vi "List Info by Socket.vi"(7 "Socket":u32, 11 "LookupTable":refnum<data-value>) -> (3 "Pin Info":T1[](array[typedef]))   [LabVIEW 2024, in "Shared Steps.lvlib"]
doc: "Helper Routine: List all pins for a given socket."
uses:
  Shared Steps.lvlib
  Types/Pin Mapping.ctl
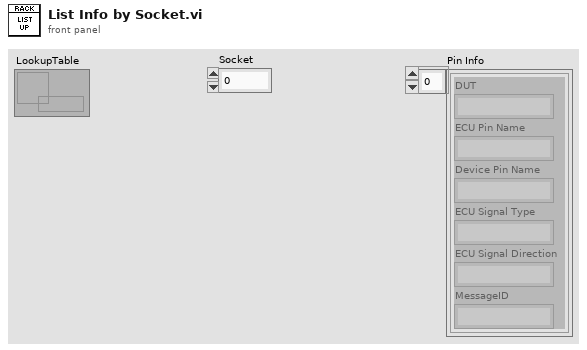
[diagram p1: front panel]
types:
  T1 = typedef "Shared Steps.lvlib/Pin Mapping.ctl" = cluster{"DUT":string, "ECU Pin Name":string, "Device Pin Name":string, "ECU Signal Type":string, "ECU Signal Direction":string, "MessageID":string}
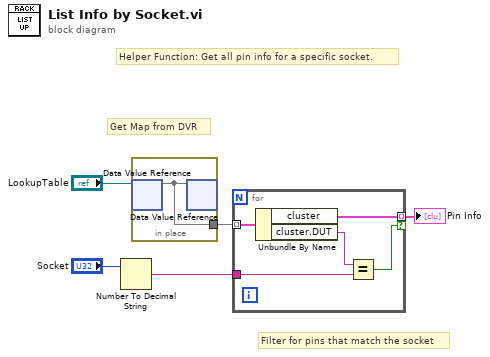
[diagram p0: block diagram]
diagram:
  # "Filter for pins that match the socket"
  # "Get Map from DVR"
  # "Helper Function: Get all pin info for a specific socket."
  n1 = Number To Decimal String(number="Socket") -> (decimal integer string=w2:string)  [unwired: 1 in]
  n2 = in-place {
    in-place-border: [w6] -> w4
    n3 = in-place-dvr #1("LookupTable") -> (w6:map{string, T1})  [unwired: 1 out]
    n4 = in-place-dvr #1(w6) -> ()  [unwired: 2 out]
  }
  n5 = for {
    tunnel: w4 -> [w11] mode=indexing
    tunnel: w2 -> [w9]
    tunnel: [w8] -> w1 mode=indexing if=w7
    n6 = Unbundle By Name(w11) -> ("cluster"=w8:T1, "cluster.DUT"=w10:string)
    n7 = Equal?(x=w10, y=w9) -> (x = y?=w7:bool)
  }
  "Pin Info" <- w1
